vi "Write Meta Data (TCP Ref).vi"(6 "options":T1={"ignore timeout error"=TRUE, "timeout ms (1000)"=1000}, 7 "meta data":T2[](array[typedef]), 8 "error in":errorcluster, 11 "connection ID":refnum<k5>) -> (0 "error out":errorcluster, 3 "connection info out":T3)   [LabVIEW 2013, in "NI STM.lvlib"]
doc: "Use this VI to transmit the meta data cluster to a remote computer. Sending the meta data to another computer helps maintainability since the data resides only on one side and it is shared to other computers at run time."
uses:
  NI STM.lvlib
  TCP Connection Info.ctl
  SubVIs/MetaDataElement.ctl
  TCP Write Options.ctl
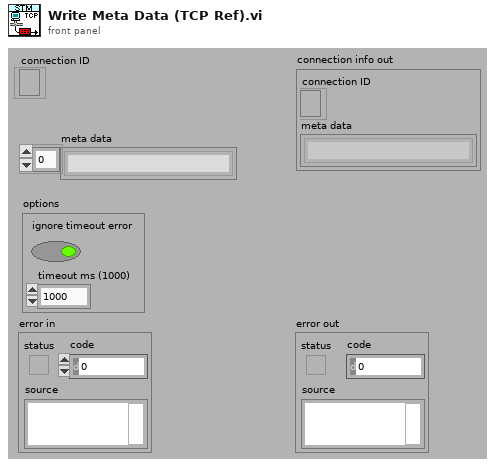
[diagram p1: front panel]
types:
  T1 = typedef "NI STM.lvlib/TCP Write Options.ctl" = cluster{"ignore timeout error":bool, "timeout ms (1000)":i32}
  T2 = typedef "NI STM.lvlib/MetaDataElement.ctl" = string
  T3 = typedef "NI STM.lvlib/TCP Connection Info.ctl" = cluster{"connection ID":refnum<k5>, "meta data":T2[]}
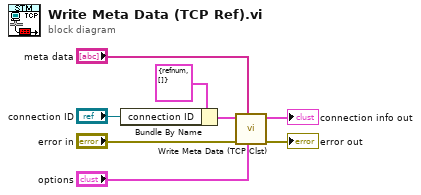
[diagram p0: block diagram]
diagram:
  n1 = Bundle By Name(cluster=T3 {"connection ID"=refnum, "meta data"=[]} ("Connection Info Out"), "connection ID"="connection ID") -> (w6:T3)
  n2 = call "Write Meta Data (TCP Clst).vi"("options"="options", "meta data"="meta data", "error in"="error in", "connection info in"=w6) -> ("error out"=→"error out":errorcluster, "connection info out"=→"connection info out":T3)  [unwired: 6 in]
